vi "7831RDIO.vi"() -> (3 "SPI DIO Lines":T1={"SCLK"="Connector0/DIO0", "MISO"="Connector0/DIO1", "MOSI"="Connector0/DIO2", "CS 0"="Connector0/DIO3", "CS 1"="Connector0/DIO3", "CS 2"="Connector0/DIO3", "CS 3"="Connector0/DIO3", "CS 4"="Connector0/DIO3", "CS 5"="Connector0/DIO3"})   [LabVIEW 2014]
uses:
  <vilib>/SPI API/SPIAPI/DIO/SPI Digital IO Lines.ctl
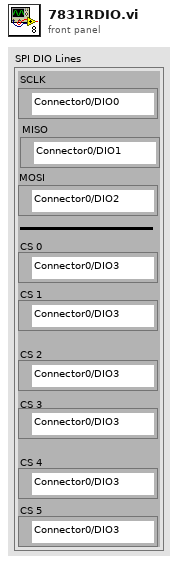
[diagram p1: front panel]
types:
  T1 = typedef "SPI Digital IO Lines.ctl" = cluster{"SCLK":refnum<k21>, "MISO":refnum<k21>, "MOSI":refnum<k21>, "CS 0":refnum<k21>, "CS 1":refnum<k21>, "CS 2":refnum<k21>, "CS 3":refnum<k21>, "CS 4":refnum<k21>, "CS 5":refnum<k21>}
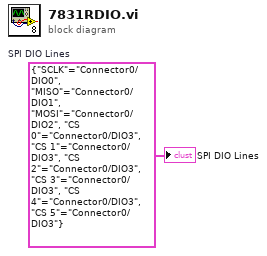
[diagram p0: block diagram]
diagram:
  w1 = T1 {"SCLK"="Connector0/DIO0", "MISO"="Connector0/DIO1", "MOSI"="Connector0/DIO2", "CS 0"="Connector0/DIO3", "CS 1"="Connector0/DIO3", "CS 2"="Connector0/DIO3", "CS 3"="Connector0/DIO3", "CS 4"="Connector0/DIO3", "CS 5"="Connector0/DIO3"}  # SPI DIO Lines
  "SPI DIO Lines" <- w1
